vi "导通电阻测试.vi"(6 "error in (no error)":errorcluster, 7 "接触电阻判断阈值":dbl[](array[numeric]), 8 "输入电流":dbl=200.0 format="%#_13g", 9 "仪器实例 in":T1) -> (0 "error out":errorcluster, 1 "x <= y?":bool[](array[boolean]), 2 "导通电阻":dbl[](array[numeric]), 3 "仪器实例 out":T1)   [LabVIEW 2020]
uses:
  F:/F020/S7_1200 control/HslCommunication.dll
  S7_1200 control/HslCommunication.dll
  S7_1200 control/S7_1200 WriteBool.vi
  <instrlib>/Keithley 27XX/Public/Data/Read Multiple Direct.vi
  <instrlib>/Keithley 27XX/Keithley 27XX.lvlib
  S7_1200 control/S7_1200 control.lvlib
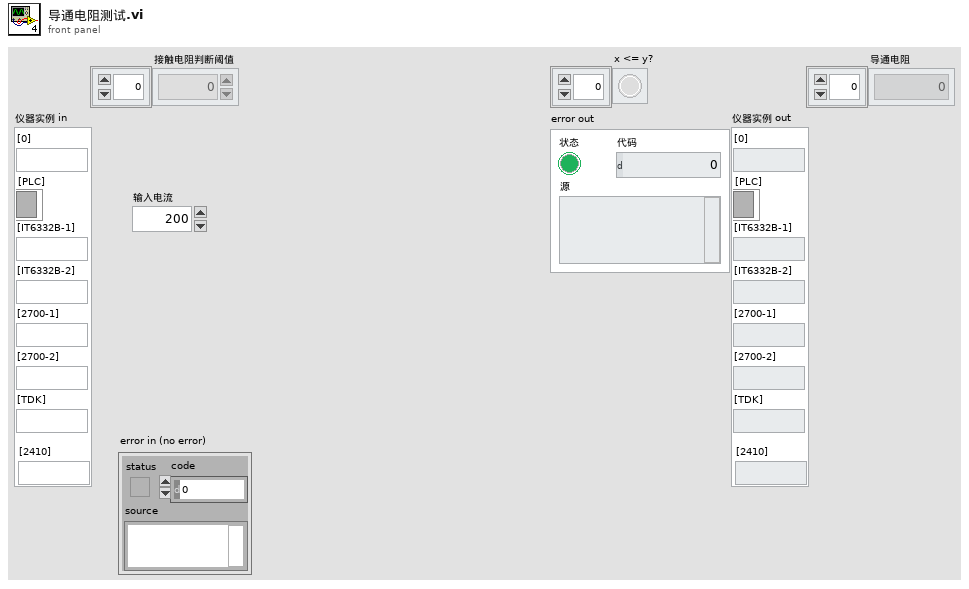
[diagram p1: front panel]
types:
  T1 = typedef "仪器实例.ctl" = cluster{"[0]":string, "[PLC]":refnum<k24>, "[IT6332B-1]":string, "[IT6332B-2]":string, "[2700-1]":string, "[2700-2]":string, "[TDK]":string, "[2410]":string}
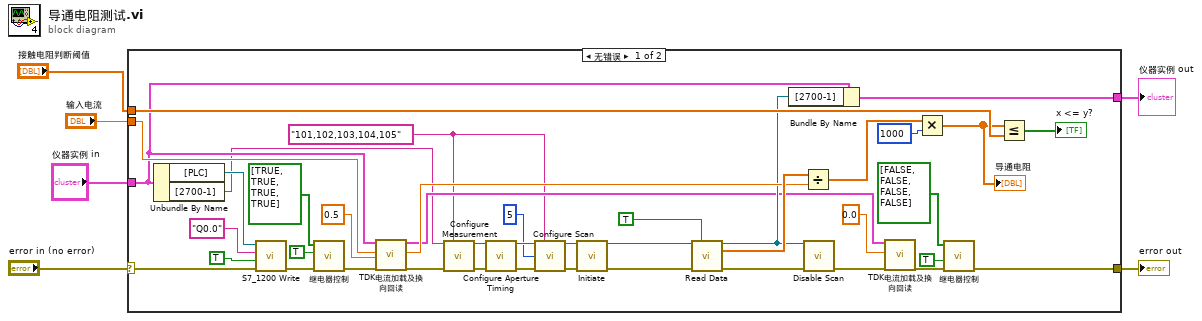
[diagram p0: block diagram]
diagram:
  n1 = case shown="无错误" "error in (no error)" {
    selector: "error in (no error)" -> [w24 w49]
    tunnel: "仪器实例 in" -> [w22 w48]
    tunnel: "输入电流" -> [w43 _]
    tunnel: "接触电阻判断阈值" -> [w40 _]
    tunnel: [w27 w49] -> w3
    tunnel: [w35 w48] -> w1
    frame No Error {
      w16 = "101,102,103,104,105" ("Scan List (Empty)")
      n2 = Unbundle By Name(w22) -> ("[PLC]"=w21:refnum<k24>, "[2700-1]"=w20:string)
      n3 = call-poly "S7_1200 Write.vi"("错误输入（无错误）"=w24, "value"=TRUE, "address"="Q0.0", "引用"=w21) -> ("错误输出"=w23:errorcluster)  [unwired: 2 in, 1 out]
      n4 = call "继电器控制.vi"("error in"=w23, "初始化"=TRUE, "继电器控制"=bool[] [TRUE, TRUE, TRUE, TRUE]) -> ("error out"=w34:errorcluster)  [unwired: 8 in]
      n5 = call "TDK电流加载及换向回读.vi"("仪器实例 in"=w22, "输入电流"=w43, "Delay Time (s)"=0.5, "error in"=w34) -> ("仪器实例 out"=w32:T1, "实际电流"=w41:dbl, "error out"=w38:errorcluster)  [unwired: 13 in]
      n6 = call <instrlib>:"Configure Measurement.vi"("VISA resource name"=w20, "Scan List (Empty)"=w16, "error in (no error)"=w38) -> ("VISA resource name out"=w15:refnum<visa-resource-name>, "error out"=w10:errorcluster)  [unwired: 11 in]
      n7 = call <instrlib>:"Configure Aperture Timing.vi"("VISA resource name"=w15, "error in (no error)"=w10) -> ("VISA resource name out"=w14:refnum<visa-resource-name>, "error out"=w11:errorcluster)  [unwired: 12 in]
      n8 = call <instrlib>:"Configure Scan.vi"("VISA resource name"=w14, "Channel List (101:110)"=w16, "Sample Count (100)"=5, "error in (no error)"=w11) -> ("VISA resource name out"=w13:refnum<visa-resource-name>, "error out"=w12:errorcluster)  [unwired: 10 in]
      n9 = call <instrlib>:"Initiate.vi"("VISA resource name"=w13, "error in (no error)"=w12) -> ("VISA resource name out"=w47:refnum<visa-resource-name>, "error out"=w46:errorcluster)  [unwired: 12 in]
      n10 = call-poly <instrlib>:"Read Data.vi"("VISA resource name"=w47, "All Data Elements (False)"=TRUE, "error in (no error)"=w46) -> ("VISA resource name out"=w37:refnum<visa-resource-name>, "Measurement Data"=w42:dbl[], "error out"=w36:errorcluster)  [unwired: 7 in, 3 out]
      n11 = Bundle By Name(cluster=w22, "[2700-1]"=w37) -> (w35:T1)
      n12 = Divide(x=w42, y=w41) -> (x/y=w19:dbl[])
      n13 = call <instrlib>:"Disable Scan.vi"("VISA resource name"=w37, "error in (no error)"=w36) -> ("error out"=w28:errorcluster)  [unwired: 12 in, 1 out]
      n14 = call "TDK电流加载及换向回读.vi"("仪器实例 in"=w32, "输入电流"=0.0, "error in"=w28) -> ("error out"=w30:errorcluster)  [unwired: 14 in, 2 out]
      n15 = Multiply(x=w19, y=1000) -> (x*y=w17:dbl[])
      "导通电阻" <- w17
      n16 = call "继电器控制.vi"("error in"=w30, "释放"=TRUE, "继电器控制"=bool[] [FALSE, FALSE, FALSE, FALSE]) -> ("error out"=w27:errorcluster)  [unwired: 8 in]
      n17 = Less Or Equal?(x=w17, y=w40) -> (x <= y?=→"x <= y?":bool[])
    }
    frame Error {
    }
  }
  "error out" <- w3
  "仪器实例 out" <- w1
